vi "index of clicked element.vi"(6 "Control cords":T1, 9 "Index Values":u32[](array[numeric]), 11 "Mouse cords":T1) -> (2 "element index":i32)   [LabVIEW 2009]
uses:
  <vilib>/Utility/miscctls.llb/LVPoint32TypeDef.ctl
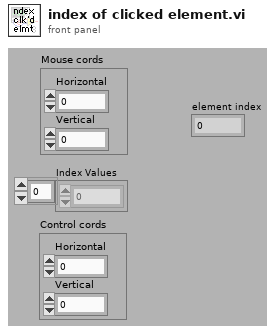
[diagram p1: front panel]
types:
  T1 = typedef "LVPoint32TypeDef.ctl" = cluster{"Horizontal":i32, "Vertical":i32}
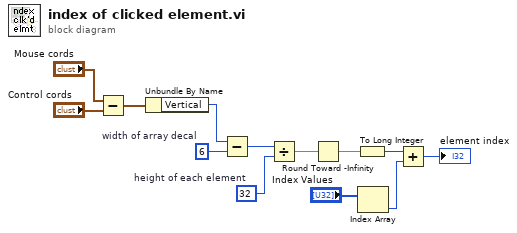
[diagram p0: block diagram]
diagram:
  w8 = 6  # width of array decal
  w6 = 32  # height of each element
  n1 = Subtract(x="Mouse cords", y="Control cords") -> (x-y=w3:T1)
  n2 = Unbundle By Name(w3) -> ("Vertical"=w9:i32)
  n3 = Subtract(x=w9, y=w8) -> (x-y=w7:i32)
  n4 = Divide(x=w7, y=w6) -> (x/y=w11:dbl)
  n5 = Round Toward -Infinity(1:w11) -> (0:w1:dbl)
  n6 = To Long Integer(number=w1) -> (32bit integer=w2:i32)
  n7 = Index Array(array="Index Values") -> (element=w12:u32)  [unwired: 1 in]
  n8 = Add(x=w2, y=w12) -> (x+y=→"element index":u32)
